vi "GET_Zone_number_(online).vi"(2 "Size of the image (480x480)":T2={"Numeric Control"=480.0, "Numeric Control"=480.0}, 3 "Mouse drawing parameters":T1, 4 "Array of the pixel to zone correspondences":T3, 5 "Animal coordinates in":T4) -> (0 "Zone":i8, 1 "Animal coordinates out":T4)   [LabVIEW 2018, in "Tracker.lvlib"]
uses:
  Tracker.lvlib
  Controls/CTL_Animal_Coordinates_and_Speed.ctl
  Controls/CTL_Pixel_to_Zone_array.ctl
  Controls/CTL_Mouse_Draw_Params.ctl
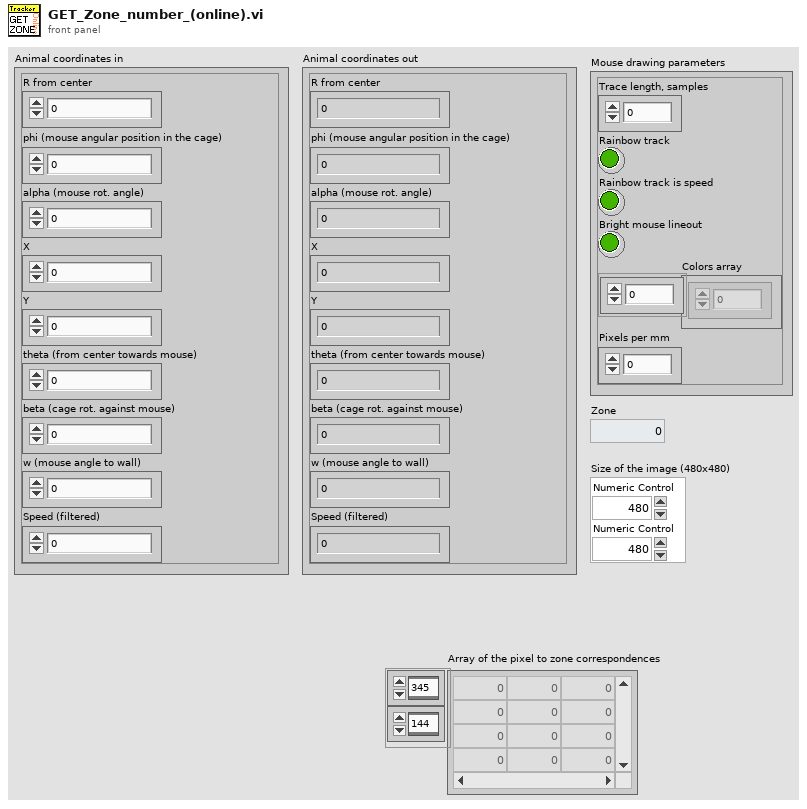
[diagram p1: front panel]
types:
  T1 = typedef "Tracker.lvlib/CTL_Mouse_Draw_Params.ctl" = cluster{"Trace length, samples":u16, "Rainbow track":bool, "Rainbow track is speed":bool, "Bright mouse lineout":bool, "Colors array":u32[], "Pixels per mm":dbl}
  T2 = cluster{"Numeric Control":dbl, "Numeric Control":dbl}
  T3 = typedef "Tracker.lvlib/CTL_Pixel_to_Zone_array.ctl" = i8[][]
  T4 = typedef "Tracker.lvlib/CTL_Animal_Coordinates_and_Speed.ctl" = cluster{"R from center":dbl, "phi (mouse angular position in the cage)":dbl, "alpha (mouse rot. angle)":dbl, "X":dbl, "Y":dbl, "theta (from center towards mouse)":dbl, "beta (cage rot. against mouse)":dbl, "w (mouse angle to wall)":dbl, "Speed (filtered)":dbl}
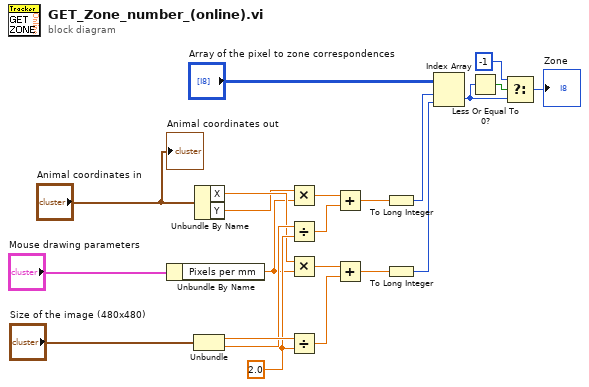
[diagram p0: block diagram]
diagram:
  w18 = 2.0
  n1 = Unbundle By Name("Mouse drawing parameters") -> ("Pixels per mm"=w12:dbl)
  n2 = Unbundle("Size of the image (480x480)") -> ("Numeric Control"=w20:dbl, "Numeric Control"=w19:dbl)
  n3 = Unbundle By Name("Animal coordinates in") -> ("X"=w14:dbl, "Y"=w13:dbl)
  n4 = Multiply(x=w13, y=w12) -> (x*y=w10:dbl)
  n5 = Divide(x=w19, y=w18) -> (x/y=w16:dbl)
  n6 = Multiply(x=w14, y=w12) -> (x*y=w11:dbl)
  n7 = Divide(x=w20, y=w18) -> (x/y=w17:dbl)
  n8 = Add(x=w10, y=w16) -> (x+y=w7:dbl)
  n9 = Add(x=w11, y=w17) -> (x+y=w9:dbl)
  n10 = To Long Integer(number=w7) -> (32bit integer=w5:i32)
  n11 = To Long Integer(number=w9) -> (32bit integer=w6:i32)
  n12 = Index Array(array="Array of the pixel to zone correspondences", index (row)=w5, index (col)=w6) -> (element=w1:i8)
  n13 = Less Or Equal To 0?(x=w1) -> (x <= 0?=w4:bool)
  n14 = Select(t=i8 -1, s=w4, f=w1) -> (s? t:f=→"Zone":i8)
  "Animal coordinates out" <- "Animal coordinates in"
